vi "SaveStriptestRecoveryFiles.vi"(3 "Array Titles":string, 4 "Strip Segment":string, 5 "Humidity":dbl, 6 "Temperature":dbl, 7 "Region #":u32) -> (0 "Path + Filename OUT":string, 1 "Filename OUT":string)   [LabVIEW 2019]
uses:
  general_VIs/globals/QC_RunInformation.vi
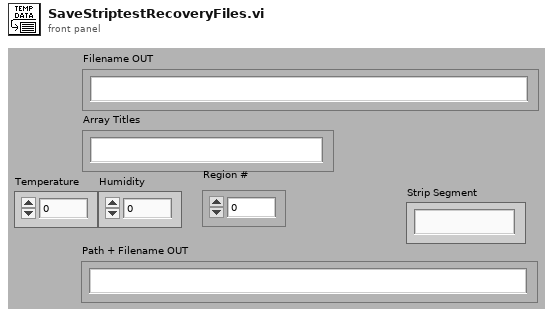
[diagram p1: front panel]
types:
  T1 = enum16{"open", "open or create", "create or replace", "create"}
  T2 = cluster{"Institute":string, "Manufacturers":string[], "Devices":string[], "Serialnumbers Lookup DB":string, "Data directory":string, "Backup & screenshot directory":string, "List of known users":string[], "Measurement switch not used":bool, "Measurement Switch":string, "DUT Switch":string}
  T3 = enum16{"Reset", "Read Array", "Read Element", "Write Element", "Write Array", "Add Element", "Add Array"}
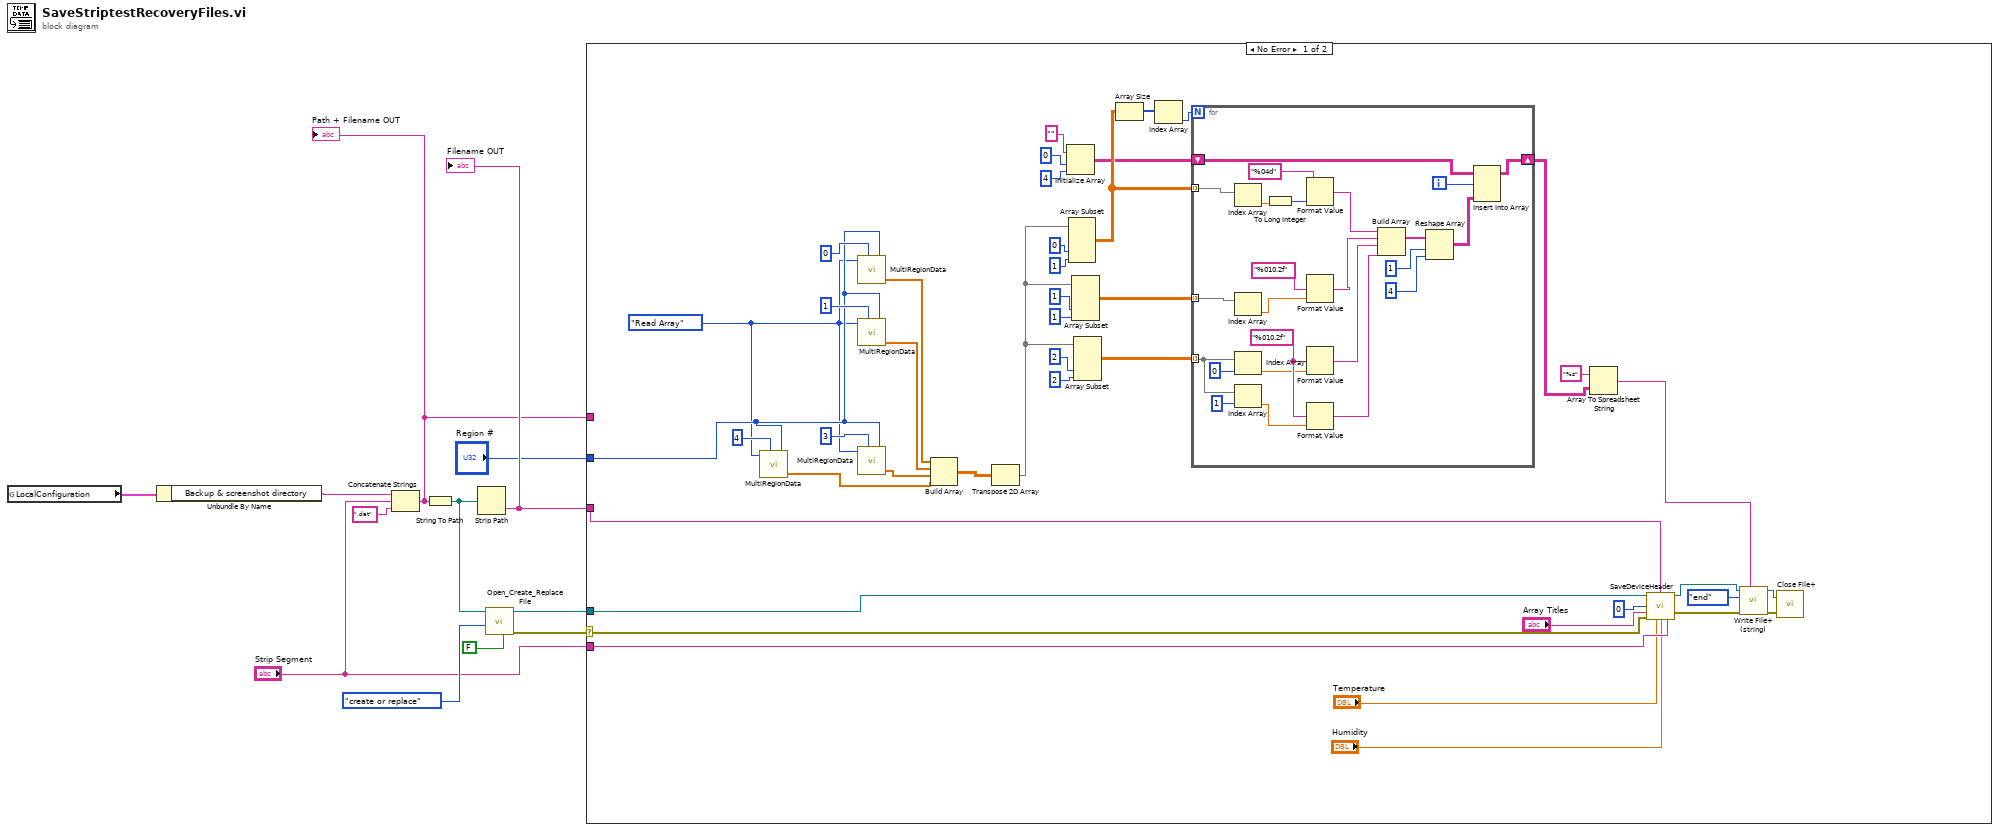
[diagram p0: block diagram]
diagram:
  n1 = global read "QC_RunInformation.vi" "LocalConfiguration"() -> (w4:T2)
  n2 = Unbundle By Name(w4) -> ("Backup & screenshot directory"=w3:string)
  n3 = Concatenate Strings(w3, "Strip Segment", ".dat") -> (w6:string)
  "Path + Filename OUT" <- w6
  n4 = String To Path(string=w6) -> (path=w9:path)
  n5 = Strip Path(path=w9) -> (name=w10:string)  [unwired: 1 out]
  "Filename OUT" <- w10
  n6 = call <vilib>:"Open_Create_Replace File.vi"("advisory dialog? (display:T)"=FALSE, "function (open:0)"=T1."create or replace", "file path"=w9) -> ("error out"=w8:errorcluster, "refnum"=w11:refnum<file>)  [unwired: 5 in, 2 out]
  n7 = case shown="No Error" w8 {
    selector: w8 -> [w55 _]
    tunnel: w11 -> [w52 _]
    tunnel: w6 -> [_ _]
    tunnel: w10 -> [w53 _]
    tunnel: "Region #" -> [w41 _]
    tunnel: "Strip Segment" -> [w38 _]
    frame No Error {
      w36 = T3."Read Array" ("Action")
      n8 = call "MultiRegionData.vi"("Action"=w36, "Array No."=4, "Region index"=w41) -> ("Array OUT"=w34:dbl[])  [unwired: 3 in, 1 out]
      n9 = call "MultiRegionData.vi"("Action"=w36, "Array No."=0, "Region index"=w41) -> ("Array OUT"=w43:dbl[])  [unwired: 3 in, 1 out]
      n10 = call "MultiRegionData.vi"("Action"=w36, "Array No."=1, "Region index"=w41) -> ("Array OUT"=w44:dbl[])  [unwired: 3 in, 1 out]
      n11 = call "MultiRegionData.vi"("Action"=w36, "Array No."=3, "Region index"=w41) -> ("Array OUT"=w35:dbl[])  [unwired: 3 in, 1 out]
      n12 = Build Array(w43, w44, w35, w34) -> (w42:dbl[][])
      n13 = Transpose 2D Array(2D array=w42) -> (transposed array=w16:dbl[][])
      n14 = Initialize Array("", 0 ("dimension size"), 4 ("dimension size")) -> (w19:string[][])
      n15 = Array Subset(array=w16, index (col)=0 ("index"), length (col)=1 ("length")) -> (w22:dbl[][])  [unwired: 2 in]
      n16 = Array Subset(array=w16, index (col)=1 ("index"), length (col)=1 ("length")) -> (w24:dbl[][])  [unwired: 2 in]
      n17 = Array Subset(array=w16, index (col)=2 ("index"), length (col)=2 ("length")) -> (w23:dbl[][])  [unwired: 2 in]
      n18 = Array Size(array=w22) -> (size(s)=w21:i32[])
      n19 = Index Array(array=w21) -> (element=w20:i32)  [unwired: 1 in]
      n20 = for {
        N: w20 -> [_]
        tunnel: w24 -> [w72] mode=indexing
        tunnel: w23 -> [w75] mode=indexing
        tunnel: w22 -> [w73] mode=indexing
        shift-right: [w78] -> w17
        shift-left: w19 -> [w77]
        i -> [w79]
        w66 = "%010.2f" ("format string")
        n21 = Index Array(array=w73) -> (element=w70:dbl)  [unwired: 1 in]
        n22 = Index Array(array=w72) -> (element=w68:dbl)  [unwired: 1 in]
        n23 = Index Array(array=w75, index=0) -> (element=w65:dbl)
        n24 = Index Array(array=w75, index=1) -> (element=w64:dbl)
        n25 = To Long Integer(number=w70) -> (32bit integer=w71:i32)
        n26 = Format Value(format string="%04d", value (0)=w71) -> (output string=w63:string)  [unwired: 1 in]
        n27 = Format Value(format string="%010.2f", value (0)=w68) -> (output string=w62:string)  [unwired: 1 in]
        n28 = Format Value(format string=w66, value (0)=w65) -> (output string=w61:string)  [unwired: 1 in]
        n29 = Format Value(format string=w66, value (0)=w64) -> (output string=w60:string)  [unwired: 1 in]
        n30 = Build Array(w63, w62, w61, w60) -> (w59:string[])
        n31 = Reshape Array(w59, 1 ("dimension size"), 4 ("dimension size")) -> (w56:string[][])
        n32 = Insert Into Array(array=w77, index (row)=w79, new element=w56) -> (w78:string[][])  [unwired: 1 in]
      }
      n33 = Array To Spreadsheet String(array=w17, 3:"%s" ("format string")) -> (spreadsheet string=w15:string)  [unwired: 1 in]
      n34 = call "SaveDeviceHeader.vi"("File Refnum in"=w52, "Filename"=w53, "Run Number"=0, "Array Titles"="Array Titles", "error in (no error)"=w55, "Temperature"="Temperature", "Humidity"="Humidity", "Strip Structure"=w38) -> ("File Refnum out"=w40:refnum<file>, "error out"=w39:errorcluster)  [unwired: 5 in, 1 out]
      n35 = call <vilib>:"Write File+ (string).vi"("string"=w15, "error in (no error)"=w39, "pos mode (rel. to end:1)"=enum16{"start", "end", "current"}."end", "refnum"=w40) -> ("error out"=w50:errorcluster, "dup refnum"=w51:refnum<file>)  [unwired: 3 in, 1 out]
      n36 = call <vilib>:"Close File+.vi"("error in (no error)"=w50, "refnum"=w51) -> ()  [unwired: 3 in, 3 out]
    }
    frame Error {
    }
  }
